vi "Set Visibility.vi"(8 "error in (no error)":errorcluster, 9 "Show Progress":bool=TRUE, 10 "Visible?":bool=TRUE, 11 "Viewer in":refnum<class "Viewer.lvclass">) -> (0 "error out":errorcluster, 3 "Viewer out":refnum<class "Viewer.lvclass">)   [LabVIEW 2023, in "Viewer.lvlib" / "Viewer.lvclass"]
uses:
  Viewer.lvclass
  <vilib>/event_ctls.llb/usereventprio.ctl
  Viewer.lvclass/Viewer.ctl
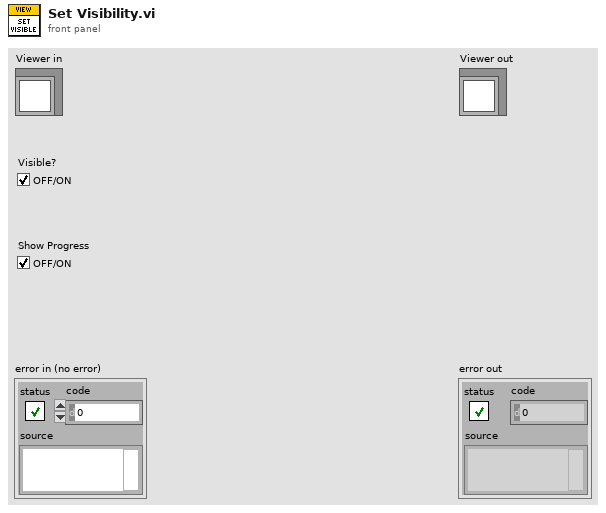
[diagram p1: front panel]
types:
  T1 = typedef "usereventprio.ctl" = enum32{"high priority", "normal priority"}
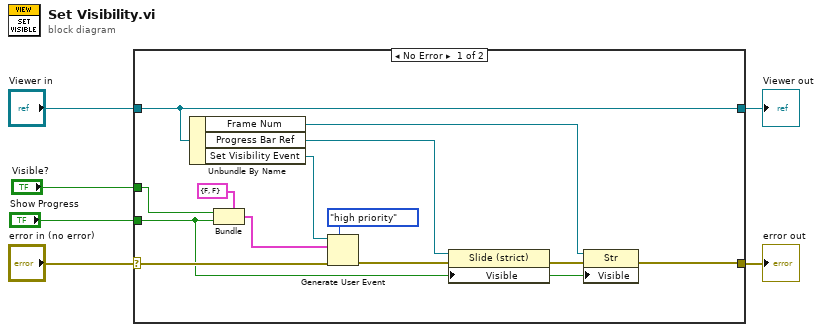
[diagram p0: block diagram]
diagram:
  n1 = case shown="No Error" "error in (no error)" {
    selector: "error in (no error)" -> [w19 w21]
    tunnel: [w9 w21] -> w5
    tunnel: [w18 w20] -> w3
    tunnel: "Viewer in" -> [w18 w20]
    tunnel: "Visible?" -> [w15 _]
    tunnel: "Show Progress" -> [w7 _]
    frame No Error {
      n2 = Unbundle By Name(w18) -> ("Frame Num"=w8:refnum<vi>, "Progress Bar Ref"=w11:refnum<vi>, "Set Visibility Event"=w17:refnum<user-event>)
      n3 = Bundle(cluster=cluster{"Visible?":bool, "Show Progress":bool} {"Visible?"=FALSE, "Show Progress"=FALSE}, "Visible?"=w15, "Show Progress"=w7) -> (w13:cluster{"Visible?":bool, "Show Progress":bool})
      n4 = Generate User Event(priority (normal)=usereventprio."high priority", user event=w17, event data cluster=w13, error in=w19) -> (error out=w12:errorcluster)  [unwired: 1 out]
      n5 = property class="Slide (strict)"(reference=w11, error in=w12, "Visible"=w7) -> (error out=w10:errorcluster)  [unwired: 1 out]
      n6 = property class="Str"(reference=w8, error in=w10, "Visible"=w7) -> (error out=w9:errorcluster)  [unwired: 1 out]
    }
    frame Error {
    }
  }
  "error out" <- w5
  "Viewer out" <- w3
